vi "Convert DDS Cluster values (dBm to level).vi"(1 "DDS Values (power in dBm)":T1) -> (0 "DDS Values (power is a level)":T1)   [LabVIEW 2010]
uses:
  Controls and Type Defs/Novatech Params Type Def.ctl
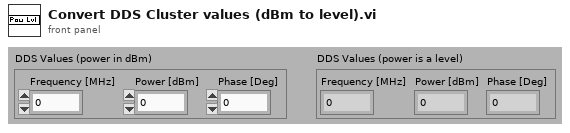
[diagram p1: front panel]
types:
  T1 = typedef "Novatech Params Type Def.ctl" = cluster{"Frequency [MHz]":dbl, "Power [dBm]":dbl, "Phase [Deg]":u16}
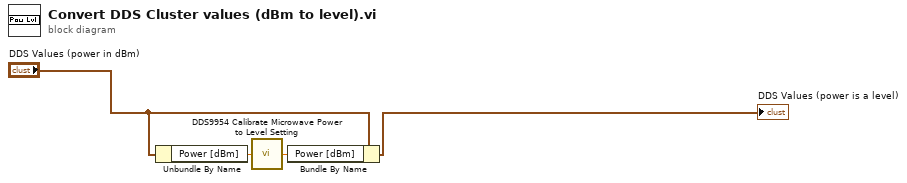
[diagram p0: block diagram]
diagram:
  n1 = Unbundle By Name("DDS Values (power in dBm)") -> ("Power [dBm]"=w1:dbl)
  n2 = call "DDS9954 Calibrate Microwave Power to Level Setting.vi"("Desired Microwave Power [dBm]"=w1) -> ("Corresponding DDS Amplitude Fraction (0-1)"=w3:dbl)  [unwired: 4 out]
  n3 = Bundle By Name(cluster="DDS Values (power in dBm)", "Power [dBm]"=w3) -> (→"DDS Values (power is a level)":T1)
